vi "IFS_Query.vi"(0 "System no.":i32=1 min=1 step=1, 2 "Interface parameter":string[](array[string]), 3 "All Parameters?":bool, 5 "error in":errorcluster) -> (14 "Parameter value":string[](array[string]), 15 "interface parameter out":string[](array[string]), 19 "error out":errorcluster)   [LabVIEW 2020]
doc: "Returns the default interface configuration which is stored in EPROM.\n\nC-887, F-206, M-8X0: Only for GCS syntax version = GCS 2.0 or higher (check with CSV?.vi. If CSV?.vi is not supported, syntax version is GCS 1.0)."
panel:
  # "Returns the default InterFace configuration which is Stored in EPROM."
  # "Query"
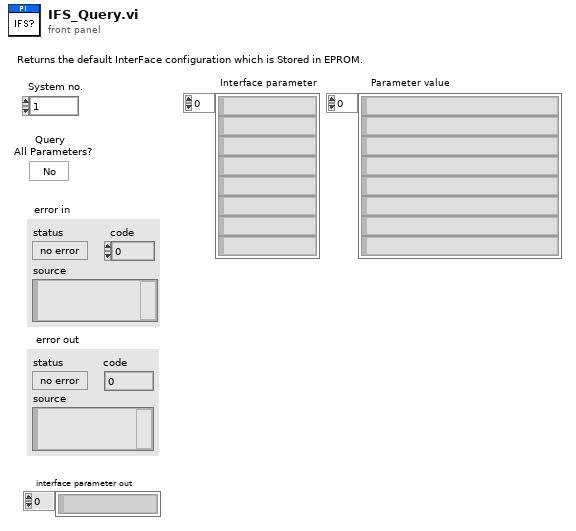
[diagram p1: front panel]
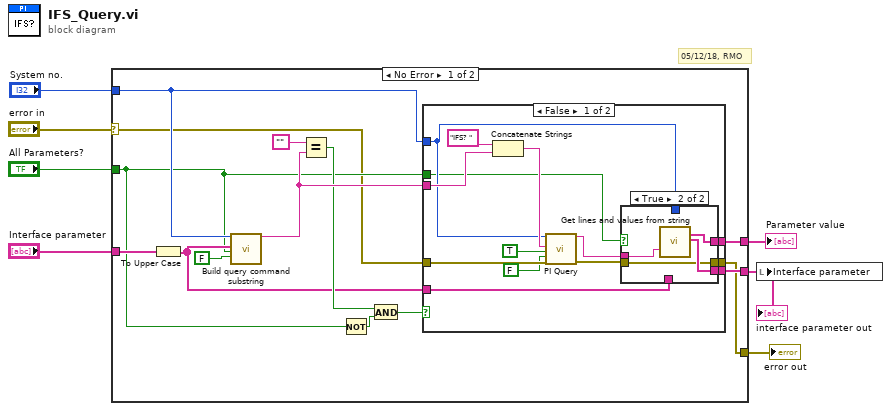
[diagram p0: block diagram]
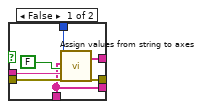
[diagram p2: hidden frame]
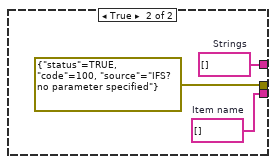
[diagram p3: hidden frame]
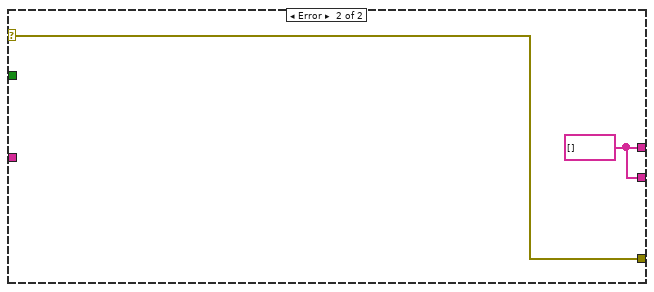
[diagram p4: hidden frame]
diagram:
  # "05/12/18, RMO"
  n1 = case shown="No Error" "error in" {
    selector: "error in" -> [w8 w50]
    tunnel: "Interface parameter" -> [w21 _]
    tunnel: [w10 w50] -> w6
    tunnel: "System no." -> [w18 _]
    tunnel: "All Parameters?" -> [w12 _]
    tunnel: [w15 w51] -> w3
    tunnel: [w11 w51] -> w2
    frame No Error {
      n2 = To Upper Case(1:w21) -> (0:w13:string[])
      n3 = call "Build query command substring.vi"("System no."=w18, "Axes to query in"=w13, "Query\nAll axes?"=w12, "For all axes: use\nAxis identifier?"=FALSE ("For all axes: use\nAxis identifier?")) -> ("Command substring"=w19:string)  [unwired: 2 in, 13 out]
      n4 = Equal?(x="", y=w19) -> (x = y?=w16:bool)
      n5 = Not(x=w12) -> (.not. x?=w17:bool)
      n6 = And(x=w16, y=w17) -> (x .and. y?=w9:bool)
      n7 = case shown="False" w9 {
        tunnel: w19 -> [w32 _]
        tunnel: w18 -> [w31 _]
        tunnel: [w30 w48] -> w15
        tunnel: w8 -> [w29 _]
        tunnel: w13 -> [w28 _]
        tunnel: w12 -> [w27 _]
        tunnel: [w26 w47] -> w11
        tunnel: [w25 errorcluster {"status"=TRUE, "code"=100, "source"="IFS? no parameter specified"} ("error out")] -> w10
        frame False {
          n8 = Concatenate Strings("IFS? ", w32) -> (w33:string)
          n9 = call "PI Query.vi"("System no."=w31, "String to send"=w33, "Attach termination char.?"=TRUE ("Attach Linefeed?"), "Strip spaces?"=FALSE, "error in"=w29) -> ("String read"=w24:string, "error out"=w22:errorcluster)  [unwired: 2 in, 11 out]
          n10 = case shown="True" w27 {
            tunnel: w31 -> [w42 _]
            tunnel: w24 -> [w41 w46]
            tunnel: [w40 w45] -> w30
            tunnel: w22 -> [w39 w43]
            tunnel: [w38 w43] -> w25
            tunnel: w28 -> [w36 _]
            tunnel: [w36 w44] -> w26
            frame False {
              n11 = call "Assign values from string to axes.vi"("System no."=w42, "Queried axes"=w36, "All axes queried?"=FALSE, "Input String"=w41, "error in"=w39) -> ("Strings"=w40:string[], "error out"=w38:errorcluster)  [unwired: 4 in, 9 out]
            }
            frame True {
              n12 = call "Get lines and values from string.vi"("Input string"=w46) -> ("Strings"=w45:string[], "Item name"=w44:string[])  [unwired: 1 in, 16 out]
            }
          }
        }
        frame True {
          w47 = string[] []  # Item name
          w48 = string[] []  # Strings
        }
      }
    }
    frame Error {
      w51 = string[] [] ("Strings")
    }
  }
  "error out" <- w6
  "Parameter value" <- w3
  "interface parameter out" <- w2
  n13 = local write "Interface parameter"(w2) -> ()
